vi "readPCObinary_new.vi"(8 "error in (no error)":errorcluster, 11 "Image Path":path=path "C:/Temp/testimage.b16") -> (0 "error out":errorcluster, 3 "Image":u16[][](graph))   [LabVIEW 2010]
doc: "This vi reads ASYST-binary files which were stored after FRAP diffusion experiments. It reads out the file-header, the message lines and 4 data arrays which may be interpreted as parameters, time, intensity and intensity (fit) - arrays. \nBefore reading the data-arrays the vi checks a valid key ID in the header.\n\nINPUT: \n-start path\n\nOUTPUT:\n-FileTemplateHeader1: first part of ASYST-Header \n [0] Number of subfiles\n [1] Size of template (Header) in bytes\n [2] Number of data records\n [3] Number of comment lines \n-message lines (STRING)\n-data 1 (array of single precision float) parameters\n-data 2 (array of single precision float) time\n-data 3 (array of single precision float) intensity\n-data 4 (array of single precision float) intensity fit\n-filesize (byte)\n\n14.05.00 Volker Kiessling"
panel:
  out "Header data":u32[](array[numeric])
  out "size(s)":i32[](array[numeric])=[260, 344]
  out "header size in byte":u32=384
  out "file size in byte":u32=179264
  in  "dialog ?":bool
  out "image (V32)":u16[][](array[numeric])
  out "position after reading":i32=179264
  out "filesize (byte)":i32=179264
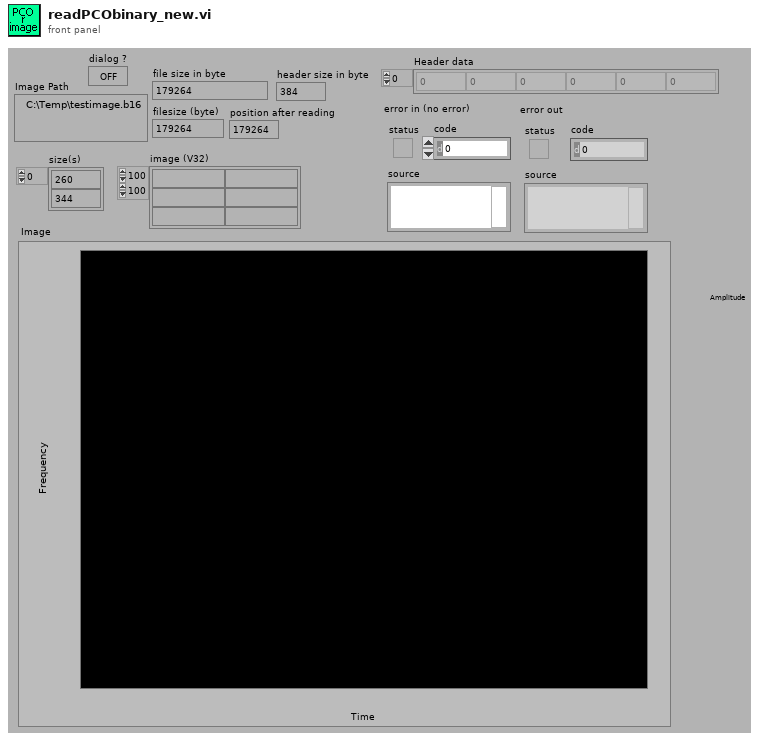
[diagram p1: front panel]
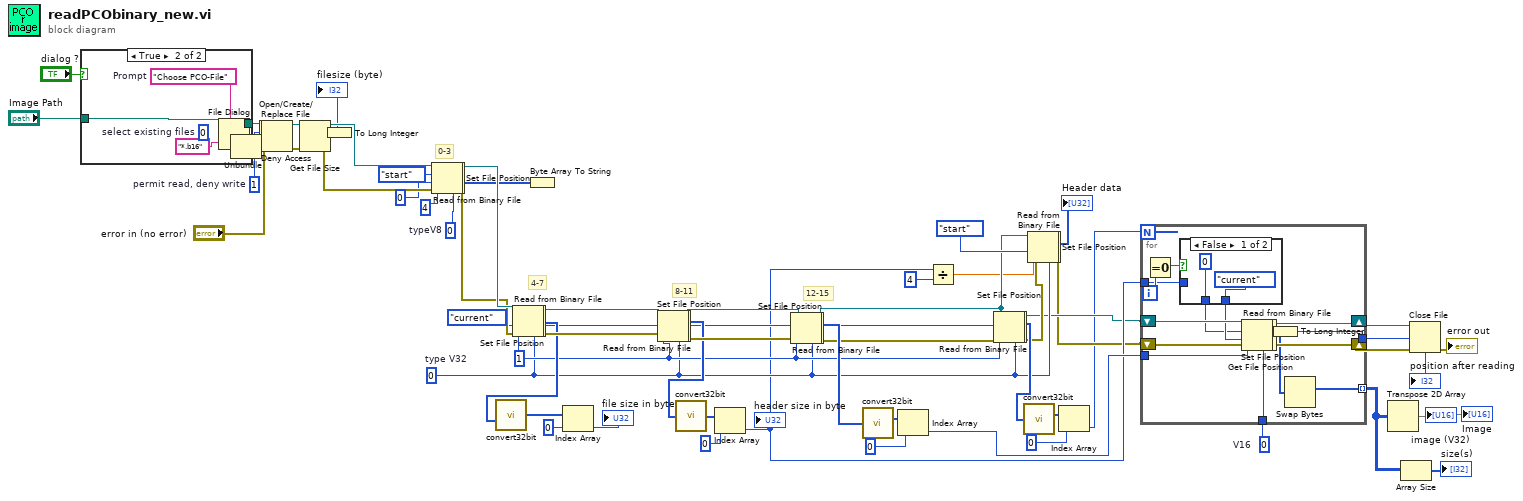
[diagram p0: block diagram]
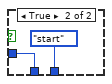
[diagram p3: hidden frame]
diagram:
  w53 = u16 0  # V16
  w39 = 1 ("count")
  w29 = u32 0  # type V32
  w40 = enum16{"start", "end", "current"}."current" ("pos mode (0:2)")
  w64 = u8 0  # typeV8
  w70 = i16 1  # permit read, deny write
  # "12-15"
  # "8-11"
  # "4-7"
  # "0-3"
  n1 = case shown="True" "dialog ?" {
    tunnel: "Image Path" -> [w73 w77]
    tunnel: [w73 w76] -> w28
    frame False {
    }
    frame True {
      w78 = "Choose PCO-File"  # Prompt
      (unwired) i16 0  # select existing files
      n2 = File Dialog(6:"*.b16" ("pattern"), 7:w78, 11:w77) -> (0:w74:errorcluster, 3:w76:path)  [unwired: 4 in, 2 out]
      n3 = Unbundle(w74) -> ()  [unwired: 3 out]
    }
  }
  n4 = Open/Create/Replace File(file path (use dialog)=w28, error in="error in (no error)") -> (refnum out=w1:refnum<file>, error out=w2:errorcluster)  [unwired: 4 in, 1 out]
  n5 = Deny Access(4:w2, 6:w70, 7:w1) -> (0:w69:errorcluster, 3:w71:refnum<file>)
  n6 = Get File Size(file=w71, error in=w69) -> (refnum out=w72:refnum<file>, size (in bytes)=w3:i64, 0:w68:errorcluster)
  n7 = To Long Integer(number=w3) -> (32bit integer=→"filesize (byte)":i32)
  n8 = Set File Position(offset (in bytes) (0)=0 ("pos offset (0)"), refnum=w72, from (0:start)=enum16{"start", "end", "current"}."start" ("pos mode (0:2)"), error in=w68) -> (refnum out=w5:refnum<file>, error out=w4:errorcluster)
  n9 = Read from Binary File(5:w64, 8:w4, 10:4 ("count"), 11:w5) -> (0:w58:errorcluster, 2:w50:u8[], 3:w62:refnum<file>)  [unwired: 2 in, 1 out]
  n10 = Set File Position(refnum=w62, from (0:start)=w40, error in=w58) -> (refnum out=w7:refnum<file>, error out=w6:errorcluster)  [unwired: 1 in]
  n11 = Read from Binary File(5:w29, 8:w6, 10:w39, 11:w7) -> (0:w57:errorcluster, 2:w46:u32[], 3:w61:refnum<file>)  [unwired: 2 in, 1 out]
  n12 = call "convert32bit.vi"("Array in"=w46) -> ("Array out"=w47:u32[])
  n13 = Byte Array To String(unsigned byte array=w50) -> ()  [unwired: 1 out]
  n14 = Index Array(array=w47, index=0 ("Index")) -> (element=→"file size in byte":u32)
  n15 = Set File Position(refnum=w61, from (0:start)=w40, error in=w57) -> (refnum out=w9:refnum<file>, error out=w8:errorcluster)  [unwired: 1 in]
  n16 = Read from Binary File(5:w29, 8:w8, 10:w39, 11:w9) -> (0:w56:errorcluster, 2:w44:u32[], 3:w59:refnum<file>)  [unwired: 2 in, 1 out]
  n17 = call "convert32bit.vi"("Array in"=w44) -> ("Array out"=w45:u32[])
  n18 = Index Array(array=w45, index=0 ("Index")) -> (element=w23:u32)
  "header size in byte" <- w23
  n19 = Set File Position(refnum=w59, from (0:start)=w40, error in=w56) -> (refnum out=w11:refnum<file>, error out=w10:errorcluster)  [unwired: 1 in]
  n20 = Read from Binary File(5:w29, 8:w10, 10:w39, 11:w11) -> (0:w33:errorcluster, 2:w41:u32[], 3:w30:refnum<file>)  [unwired: 2 in, 1 out]
  n21 = call "convert32bit.vi"("Array in"=w41) -> ("Array out"=w42:u32[])
  n22 = Index Array(array=w42, index=0 ("Index")) -> (element=w35:u32)
  n23 = Divide(x=w23, y=u32 4) -> (x/y=w25:dbl)
  n24 = Set File Position(refnum=w30, from (0:start)=w40, error in=w33) -> (refnum out=w13:refnum<file>, error out=w12:errorcluster)  [unwired: 1 in]
  n25 = Read from Binary File(5:w29, 8:w12, 10:w39, 11:w13) -> (0:w32:errorcluster, 2:w36:u32[], 3:w22:refnum<file>)  [unwired: 2 in, 1 out]
  n26 = call "convert32bit.vi"("Array in"=w36) -> ("Array out"=w38:u32[])
  n27 = Set File Position(refnum=w30, from (0:start)=enum16{"start", "end", "current"}."start" ("pos mode (0:2)"), error in=w32) -> (refnum out=w15:refnum<file>, error out=w14:errorcluster)  [unwired: 1 in]
  n28 = Read from Binary File(5:w29, 8:w14, 10:w25, 11:w15) -> (0:w21:errorcluster, 2:→"Header data":u32[])  [unwired: 2 in, 2 out]
  n29 = Index Array(array=w38, index=0 ("Index")) -> (element=w18:u32)
  n30 = for {
    N: w18 -> [_]
    shift-right: [w94] -> w54
    shift-left: w22 -> [w96]
    shift-right: [w93] -> w27
    shift-left: w21 -> [w97]
    tunnel: w53 -> [w95]
    tunnel: [w92] -> w55
    tunnel: w35 -> [w91]
    tunnel: w23 -> [w85]
    tunnel: [w84] -> w19 mode=indexing
    i -> [w88]
    n31 = Equal To 0?(x=w88) -> (x = 0?=w89:bool)
    n32 = case shown="False" w89 {
      tunnel: [enum16{"start", "end", "current"}."current" ("pos mode (0:2)") enum16{"start", "end", "current"}."start" ("pos mode (0:2)")] -> w87
      tunnel: [u32 0 w100] -> w86
      tunnel: w85 -> [_ w100]
      frame False {
      }
      frame True {
      }
    }
    n33 = Set File Position(offset (in bytes) (0)=w86, refnum=w96, from (0:start)=w87, error in=w97) -> (refnum out=w83:refnum<file>, error out=w82:errorcluster)
    n34 = Read from Binary File(5:w95, 8:w82, 10:w91, 11:w83) -> (0:w80:errorcluster, 2:w90:u16[], 3:w81:refnum<file>)  [unwired: 2 in, 1 out]
    n35 = Get File Position(4:w80, 7:w81) -> (0:w93:errorcluster, 2:w79:i64, 3:w94:refnum<file>)
    n36 = To Long Integer(number=w79) -> (32bit integer=w92:i32)
    n37 = Swap Bytes(anything=w90) -> (byte swapped=w84:u16[])
  }
  "position after reading" <- w55
  n38 = Transpose 2D Array(2D array=w19) -> (transposed array=→"image (V32)" →"Image":u16[][])
  n39 = Array Size(array=w19) -> (size(s)=→"size(s)":i32[])
  n40 = Close File(refnum=w54, error in=w27) -> (error out=→"error out":errorcluster)  [unwired: 1 out]
